vi "Get JSON Config.vi"(8 "error in (no error)":errorcluster, 11 "JSON Configuration File (.json)":path=path "C:/Users/chericks/Desktop/JSONtest/labview-grpc-query-server/jsontestfile2.json") -> (0 "error out":errorcluster, 1 "File Contents":string, 2 "JSONCluster":T1, 3 "JSON Configuration File (.json) out":path=path "C:/Users/chericks/Desktop/JSONtest/labview-grpc-query-server/jsontestfile2.json")   [LabVIEW 2019]
uses:
  JSONCluster.ctl
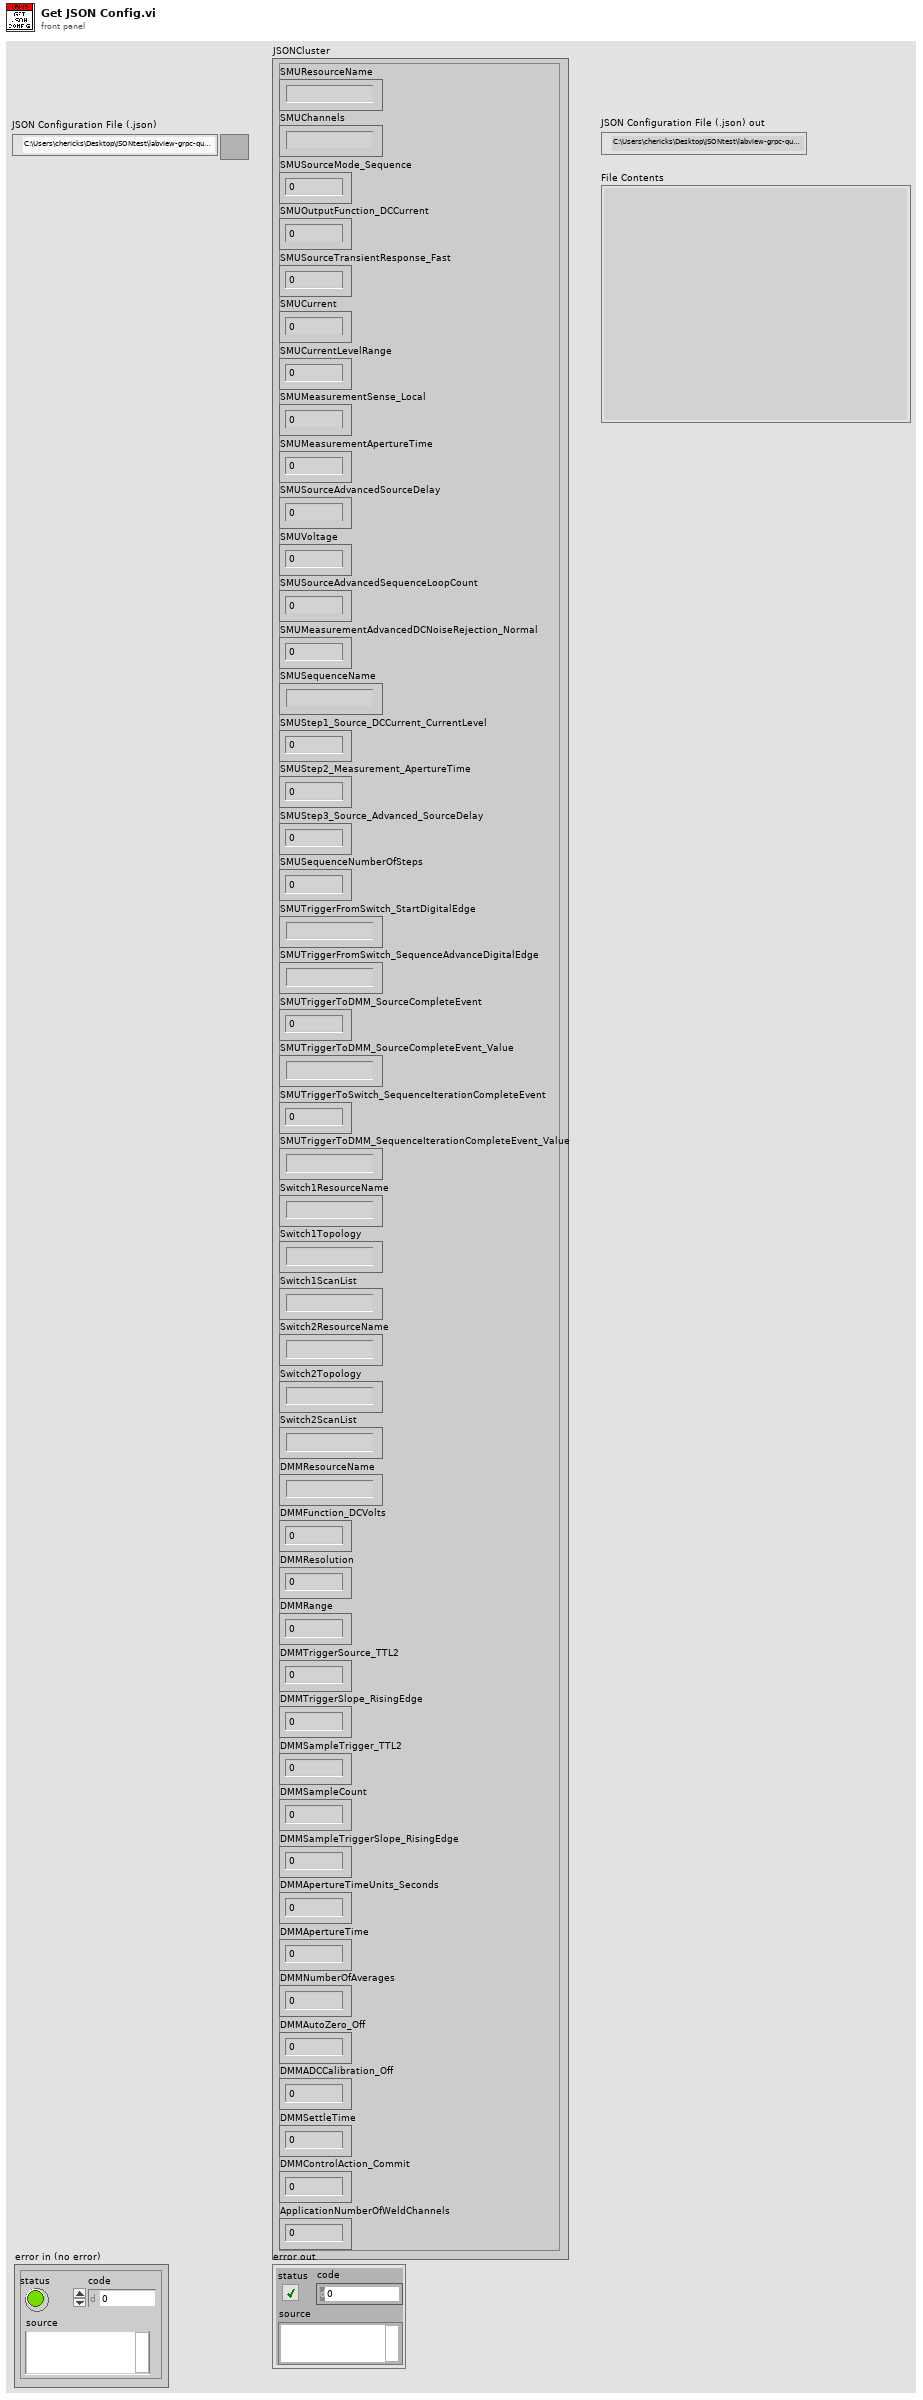
[diagram p1: front panel]
types:
  T1 = typedef "JSONCluster.ctl" = cluster{"SMUResourceName":string, "SMUChannels":string, "SMUSourceMode_Sequence":i32, "SMUOutputFunction_DCCurrent":i32, "SMUSourceTransientResponse_Fast":i32, "SMUCurrent":dbl, "SMUCurrentLevelRange":dbl, "SMUMeasurementSense_Local":i32, "SMUMeasurementApertureTime":dbl, "SMUSourceAdvancedSourceDelay":dbl, "SMUVoltage":dbl, "SMUSourceAdvancedSequenceLoopCount":i32, "SMUMeasurementAdvancedDCNoiseRejection_Normal":i32, "SMUSequenceName":string, "SMUStep1_Source_DCCurrent_CurrentLevel":i32, "SMUStep2_Measurement_ApertureTime":i32, "SMUStep3_Source_Advanced_SourceDelay":i32, "SMUSequenceNumberOfSteps":i32, "SMUTriggerFromSwitch_StartDigitalEdge":string, "SMUTriggerFromSwitch_SequenceAdvanceDigitalEdge":string, "SMUTriggerToDMM_SourceCompleteEvent":i32, "SMUTriggerToDMM_SourceCompleteEvent_Value":string, "SMUTriggerToSwitch_SequenceIterationCompleteEvent":i32, "SMUTriggerToDMM_SequenceIterationCompleteEvent_Value":string, "Switch1ResourceName":string, "Switch1Topology":string, "Switch1ScanList":string, "Switch2ResourceName":string, "Switch2Topology":string, "Switch2ScanList":string, "DMMResourceName":string, "DMMFunction_DCVolts":i32, "DMMResolution":dbl, "DMMRange":dbl, "DMMTriggerSource_TTL2":i32, "DMMTriggerSlope_RisingEdge":i32, "DMMSampleTrigger_TTL2":i32, "DMMSampleCount":i32, "DMMSampleTriggerSlope_RisingEdge":i32, "DMMApertureTimeUnits_Seconds":i32, "DMMApertureTime":dbl, "DMMNumberOfAverages":i32, "DMMAutoZero_Off":i32, "DMMADCCalibration_Off":i32, "DMMSettleTime":dbl, "DMMControlAction_Commit":i32, "ApplicationNumberOfWeldChannels":i32}
  T2 = enum16{"open", "replace", "create", "open or create", "replace or create", "replace or create with confirmation"}
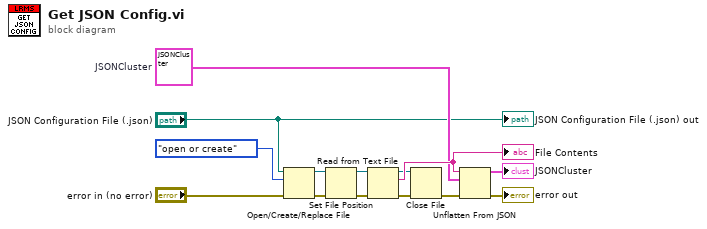
[diagram p0: block diagram]
diagram:
  w2 = T1 {"SMUResourceName"="", "SMUChannels"="", "SMUSourceMode_Sequence"=0, "SMUOutputFunction_DCCurrent"=0, "SMUSourceTransientResponse_Fast"=0, "SMUCurrent"=0.0, "SMUCurrentLevelRange"=0.0, "SMUMeasurementSense_Local"=0, "SMUMeasurementApertureTime"=0.0, "SMUSourceAdvancedSourceDelay"=0.0, "SMUVoltage"=0.0, "SMUSourceAdvancedSequenceLoopCount"=0, "SMUMeasurementAdvancedDCNoiseRejection_Normal"=0, "SMUSequenceName"="", "SMUStep1_Source_DCCurrent_CurrentLevel"=0, "SMUStep2_Measurement_ApertureTime"=0, "SMUStep3_Source_Advanced_SourceDelay"=0, "SMUSequenceNumberOfSteps"=0, "SMUTriggerFromSwitch_StartDigitalEdge"="", "SMUTriggerFromSwitch_SequenceAdvanceDigitalEdge"="", "SMUTriggerToDMM_SourceCompleteEvent"=0, "SMUTriggerToDMM_SourceCompleteEvent_Value"="", "SMUTriggerToSwitch_SequenceIterationCompleteEvent"=0, "SMUTriggerToDMM_SequenceIterationCompleteEvent_Value"="", "Switch1ResourceName"="", "Switch1Topology"="", "Switch1ScanList"="", "Switch2ResourceName"="", "Switch2Topology"="", "Switch2ScanList"="", "DMMResourceName"="", "DMMFunction_DCVolts"=0, "DMMResolution"=0.0, "DMMRange"=0.0, "DMMTriggerSource_TTL2"=0, "DMMTriggerSlope_RisingEdge"=0, "DMMSampleTrigger_TTL2"=0, "DMMSampleCount"=0, "DMMSampleTriggerSlope_RisingEdge"=0, "DMMApertureTimeUnits_Seconds"=0, "DMMApertureTime"=0.0, "DMMNumberOfAverages"=0, "DMMAutoZero_Off"=0, "DMMADCCalibration_Off"=0, "DMMSettleTime"=0.0, "DMMControlAction_Commit"=0, "ApplicationNumberOfWeldChannels"=0}  # JSONCluster
  n1 = Open/Create/Replace File(file path (use dialog)="JSON Configuration File (.json)", error in="error in (no error)", operation (0:open)=T2."open or create") -> (refnum out=w8:refnum<file>, error out=w9:errorcluster)  [unwired: 3 in, 1 out]
  n2 = Set File Position(refnum=w8, error in=w9) -> (refnum out=w6:refnum<file>, error out=w7:errorcluster)  [unwired: 2 in]
  n3 = Read from Text File(file (use dialog)=w6, error in=w7) -> (refnum out=w4:refnum<file>, text=w10:string, error out=w5:errorcluster)  [unwired: 2 in, 1 out]
  "File Contents" <- w10
  n4 = Close File(refnum=w4, error in=w5) -> (error out=w11:errorcluster)  [unwired: 1 out]
  n5 = Unflatten From JSON(JSON string=w10, type and defaults=w2, error in (no error)=w11) -> (value=→"JSONCluster":T1, error out=→"error out":errorcluster)  [unwired: 4 in]
  "JSON Configuration File (.json) out" <- "JSON Configuration File (.json)"
